vi "Update Connection Control by Reference.vi"(7 "Direction to Include":T1=enum."Publisher", 8 "error in (no error)":errorcluster, 10 "Channels":refnum<vi>, 11 "Channel Connection":refnum<vi>) -> (0 "error out":errorcluster, 2 "Channel Name":string)   [LabVIEW 2021, in "CIF_UI.lvclass"]
uses:
  CIF_UI.lvclass
  Typedef/Direction to Include.ctl
  Typedef/Channel Connection.ctl
  CIF_UI.lvclass/CIF_UI.ctl
  CIFCore/Common/CIFCoreCommon.lvlib
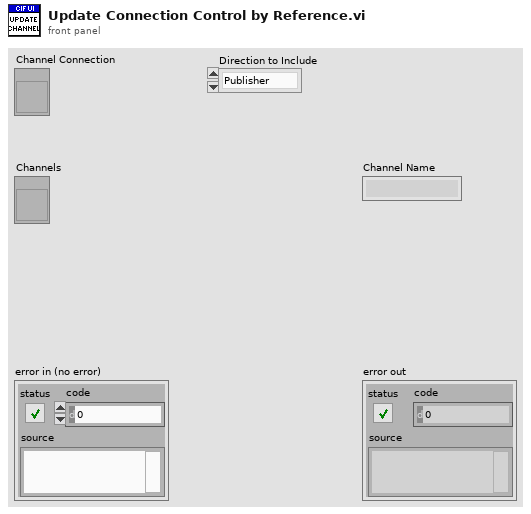
[diagram p1: front panel]
types:
  T1 = typedef "CIF_UI.lvclass/Direction to Include.ctl" = enum16{"All", "Subscriber", "Publisher"}
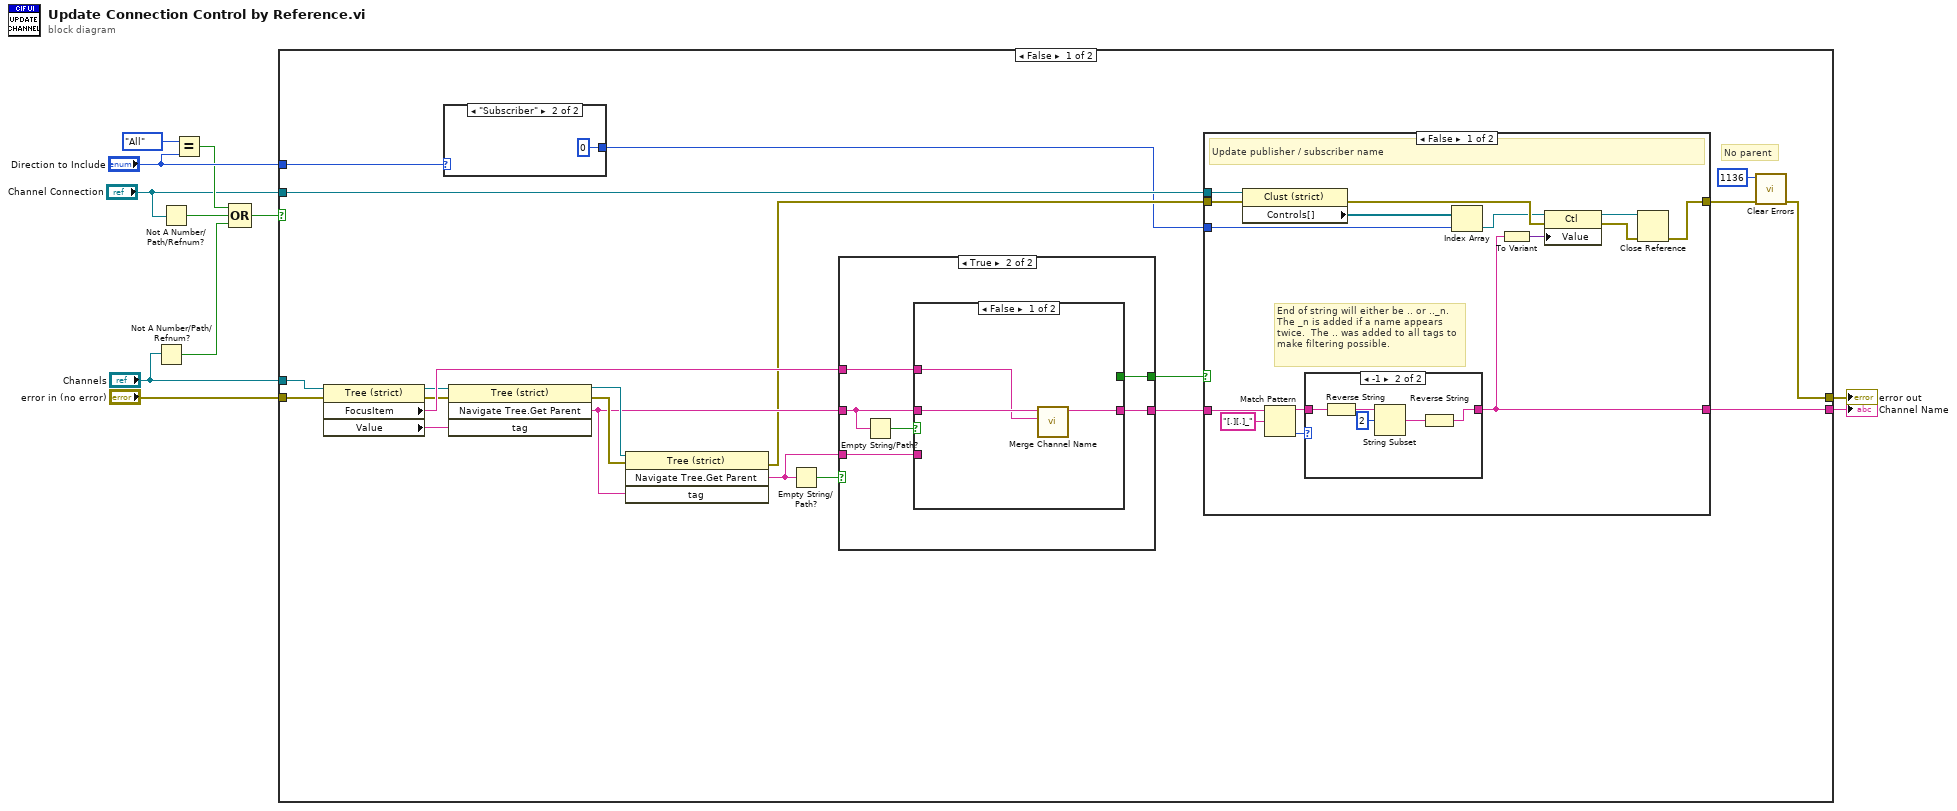
[diagram p0: block diagram]
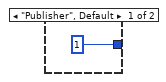
[diagram p2: hidden frame]
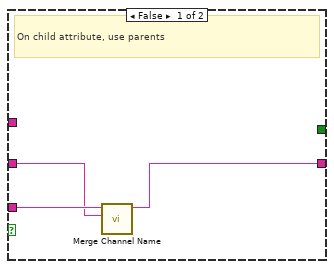
[diagram p5: hidden frame]
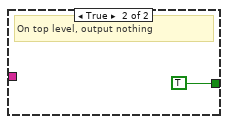
[diagram p6: hidden frame]
diagram:
  n1 = Not A Number/Path/Refnum?(number/path/refnum="Channels") -> (NaN/Path/Refnum?=w4:bool)
  n2 = Not A Number/Path/Refnum?(number/path/refnum="Channel Connection") -> (NaN/Path/Refnum?=w6:bool)
  n3 = Equal?(x=Direction_to_Include."All", y="Direction to Include") -> (x = y?=w5:bool)
  n4 = Compound Arithmetic op=OR(w5, w6, w4) -> (w3:bool)
  n5 = case shown="False" w3 {
    tunnel: "error in (no error)" -> [w26 w69]
    tunnel: [w18 w69] -> w10
    tunnel: "Channel Connection" -> [w16 _]
    tunnel: "Channels" -> [w15 _]
    tunnel: "Direction to Include" -> [w14 _]
    tunnel: [w12 _] -> w1
    frame False {
      # "No parent"
      n6 = property class="Tree (strict)"(reference=w15, error in=w26) -> (error out=w28:errorcluster, "FocusItem"=w29:string, "Value"=w31:string)  [unwired: 1 out]
      n7 = case shown="\"Subscriber\"" w14 {
        tunnel: [1 ("index") 0 ("index")] -> w13
        frame "Publisher", Default {
        }
        frame "Subscriber" {
        }
      }
      n8 = invoke class="Tree (strict)" method="Navigate Tree.Get Parent"(reference=w15, error in=w28, "tag"=w31) -> (reference out=w25:refnum<vi>, error out=w24:errorcluster, "Navigate Tree:Get Parent"=w23:string)  [unwired: 1 in, 1 out]
      n9 = invoke class="Tree (strict)" method="Navigate Tree.Get Parent"(reference=w25, error in=w24, "tag"=w23) -> (error out=w20:errorcluster, "Navigate Tree:Get Parent"=w22:string)  [unwired: 1 in, 2 out]
      n10 = Empty String/Path?(string/path=w22) -> (empty?=w30:bool)
      n11 = case shown="True" w30 {
        tunnel: w23 -> [w56 w60]
        tunnel: w29 -> [_ w61]
        tunnel: [w58 w62] -> w27
        tunnel: w22 -> [w57 w59]
        tunnel: [_ w63] -> w21
        frame False {
          # "On child attribute, use parents"
          n12 = call "Merge Channel Name.vi"("Child"=w56, "Parent"=w57) -> ("Channel Name"=w58:string)  [unwired: 9 in]
        }
        frame True {
          n13 = Empty String/Path?(string/path=w60) -> (empty?=w64:bool)
          n14 = case shown="False" w64 {
            tunnel: [_ TRUE] -> w63
            tunnel: [w67 _] -> w62
            tunnel: w61 -> [w65 _]
            tunnel: w60 -> [w66 _]
            tunnel: w59 -> [_ _]
            frame False {
              n15 = call "Merge Channel Name.vi"("Child"=w65, "Parent"=w66) -> ("Channel Name"=w67:string)  [unwired: 9 in]
            }
            frame True {
              # "On top level, output nothing"
            }
          }
        }
      }
      n16 = case shown="False" w21 {
        tunnel: w27 -> [w38 _]
        tunnel: [w47 w55] -> w19
        tunnel: w16 -> [w46 _]
        tunnel: w20 -> [w40 w55]
        tunnel: w13 -> [w39 _]
        tunnel: [w34 _] -> w12
        frame False {
          # "End of string will either be .. or .._n.  The _n is added if a name appears twice.  The .. was added to all tags to make filtering possible."
          # "Update publisher / subscriber name"
          n17 = property class="Clust (strict)"(reference=w46, error in=w40) -> (error out=w48:errorcluster, "Controls[]"=w42:refnum<vi>[])  [unwired: 1 out]
          n18 = Match Pattern(string=w38, regular expression="[.][.]_") -> (before substring=w35:string, offset past match=w36:i32)  [unwired: 1 in, 2 out]
          n19 = case shown="-1" w36 {
            tunnel: w35 -> [w49 w54]
            tunnel: [w49 w50] -> w34
            frame 0, Default {
            }
            frame -1 {
              n20 = Reverse String(1:w54) -> (0:w53:string)
              n21 = String Subset(string=w53, offset (0)=2) -> (substring=w51:string)  [unwired: 1 in]
              n22 = Reverse String(1:w51) -> (0:w50:string)
            }
          }
          n23 = Index Array(array=w42, index=w39) -> (element=w41:refnum<vi>)
          n24 = To Variant(anything=w34) -> (Variant=w45:variant)
          n25 = property class="Ctl"(reference=w41, error in=w48, "Value"=w45) -> (reference out=w44:refnum<vi>, error out=w43:errorcluster)
          n26 = Close Reference(reference=w44, error in (no error)=w43) -> (error out=w47:errorcluster)
        }
        frame True {
        }
      }
      n27 = call <vilib>:"Clear Errors.vi"("error in (no error)"=w19, "specific error code to clear (0: all)"=1136) -> ("error out"=w18:errorcluster)  [unwired: 4 in, 1 out]
    }
    frame True {
    }
  }
  "error out" <- w10
  "Channel Name" <- w1
